vi "Test All Symbols Returned.vi"(8 "error in (no error)":errorcluster, 11 "Test Case In":refnum<class "Conditional Disabled Configurator Test.lvclass">) -> (0 "error out":errorcluster, 3 "Test Case Out":refnum<class "Conditional Disabled Configurator Test.lvclass">)   [LabVIEW 2020, in "Conditional Disabled Configurator Test.lvclass"]
uses:
  Conditional Disabled Configurator Test.lvclass
  Conditional Disabled Configurator Test.lvclass/Conditional Disabled Configurator Test.ctl
  01074fa8-ee8a-411d-bc8b-fc92c4f90959.vi
  source/Conditional Disabled Configurator/Conditional Disabled Configurator.lvclass
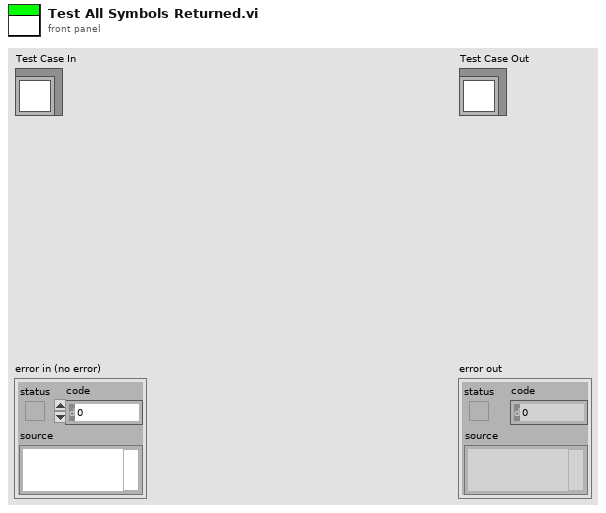
[diagram p1: front panel]
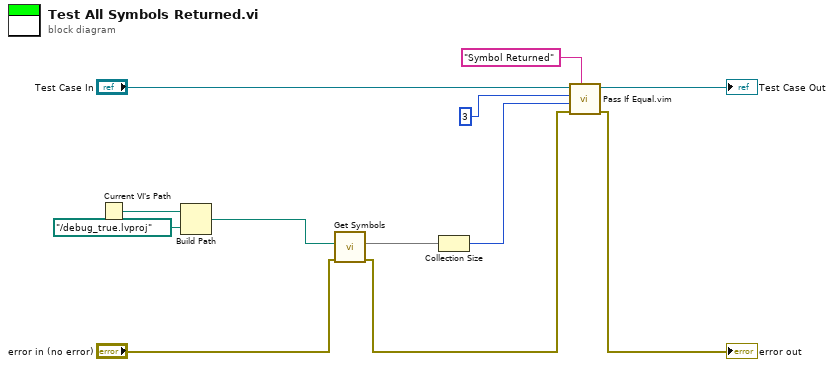
[diagram p0: block diagram]
diagram:
  n1 = Current VI's Path() -> (path=w9:path)
  n2 = Build Path(base path=w9, name or relative path=path "../debug_true.lvproj") -> (appended path=w7:path)
  n3 = call "Get Symbols.vi"("error in (no error)"="error in (no error)", "Project Path"=w7) -> ("error out"=w5:errorcluster, "Symbols"=w2:map{string, string})  [unwired: 8 in]
  n4 = Collection Size(1:w2) -> (0:w4:i32)
  n5 = call "Pass If Equal.vim"("Description"="Symbol Returned", "error in (no error)"=w5, "Actual"=w4, "Expected"=3 ("size"), "LUnit Test Case In"="Test Case In") -> ("error out"=→"error out":errorcluster, "LUnit Test Case Out"=→"Test Case Out":refnum<class "Conditional Disabled Configurator Test.lvclass">)  [unwired: 5 in]
